vi "Blink Lights.vi"(8 "error in (no error)":errorcluster, 11 "BlinkyLightModel In":refnum<class "BlinkyLightModel.lvclass">) -> (0 "error out":errorcluster, 3 "BlinkyLightModel Out":refnum<class "BlinkyLightModel.lvclass">)   [LabVIEW 2017, in "BlinkyLightModel.lvlib" / "BlinkyLightModel.lvclass"]
uses:
  <vilib>/gpm_packages/@cs/example/Dynamic Viewables/SequenceSteps/BlinkyLightModel/BlinkyLightModel.lvclass
  C:/Program Files/National Instruments/LabVIEW 2017/vi.lib/gpm_packages/@cs/mva-core/Source/IModel/IModel/IModel.lvclass
  C:/Program Files/National Instruments/LabVIEW 2017/vi.lib/ActorFramework/Actor/Actor.lvclass
  <vilib>/gpm_packages/@cs/example/Dynamic Viewables/SequenceSteps/BlinkyLightModel/BlinkyLightModel.lvclass/BlinkyLightModel.ctl
  <vilib>/gpm_packages/@cs/mva-core/Source/IObserver/IObserver/IObserver.lvclass/IObserver.ctl
  <vilib>/gpm_packages/@cs/mva-core/Source/IModel/IModel/IModel.lvclass/IModel.ctl
  <vilib>/gpm_packages/@cs/mva-core/Source/IMediator/PublishRequest/PublishRequest.lvclass/PublishRequest.ctl
  <vilib>/gpm_packages/@cs/mva-core/Source/IMediator/IMediator Messages/Publish Msg/Publish Msg.lvclass/Publish Msg.ctl
  <vilib>/gpm_packages/@cs/actor-framework-messages/Source/RoundTripMessage/RoundTripMessage.lvclass/RoundTripMessage.ctl
  <vilib>/ActorFramework/Message Enqueuer/Message Enqueuer.lvclass/Message Enqueuer.ctl
  <vilib>/ActorFramework/Actor/Actor.lvclass/Actor.ctl
  cb7bf9b9-956b-4f49-b468-f64f0c203643.vi
  <vilib>/gpm_packages/@cs/mva-core/Source/IMediator/IMediator Messages/Publish Msg/Send Pre-Addressed Publish.vi
  <vilib>/gpm_packages/@cs/mva-core/Source/IObserver/IObserver/Read Unique ID.vi
  <vilib>/gpm_packages/@cs/mva-core/Source/IMediator/PublishRequest/Pack Publish Request.vi
  <vilib>/ActorFramework/Message Enqueuer/Init from Existing Queue.vi
  <vilib>/ActorFramework/Message Enqueuer/Enqueue.vi
  <vilib>/gpm_packages/@cs/actor-framework-messages/Source/RoundTripMessage/Return Round-Trip Message.vi
  <vilib>/gpm_packages/@cs/mva-core/Source/IModel/IModel/IModel.lvclass
  C:/Program Files/National Instruments/LabVIEW 2017/vi.lib/gpm_packages/@cs/mva-core/Source/IObserver/IObserver/IObserver.lvclass
  <vilib>/gpm_packages/@cs/mva-core/Source/IMediator/IMediator Messages/Publish Msg/Publish Msg.lvclass
  C:/Program Files/National Instruments/LabVIEW 2017/vi.lib/gpm_packages/@cs/actor-framework-messages/Source/RoundTripMessage/RoundTripMessage.lvclass
  <vilib>/gpm_packages/@cs/actor-framework-messages/Source/RoundTripMessage/RoundTripMessage.lvclass
  C:/Program Files/National Instruments/LabVIEW 2017/vi.lib/ActorFramework/Message/Message.lvclass
  <vilib>/ActorFramework/Stop Msg/Stop Msg.lvclass
  <vilib>/gpm_packages/@cs/example/Dynamic Viewables/SequenceSteps/BlinkyLightModel Messages/Blink Lights Msg/Blink Lights Msg.lvclass
  <vilib>/Utility/error.llb/Error Cluster From Error Code.vi
  <vilib>/ActorFramework/Message Priority Queue/Priority Enqueue.vi
  <vilib>/gpm_packages/@cs/mva-core/Source/IMediator/PublishRequest/PublishRequest.lvclass
  <vilib>/ActorFramework/Message Enqueuer/Message Enqueuer.lvclass
  <vilib>/ActorFramework/Actor/Actor.lvclass
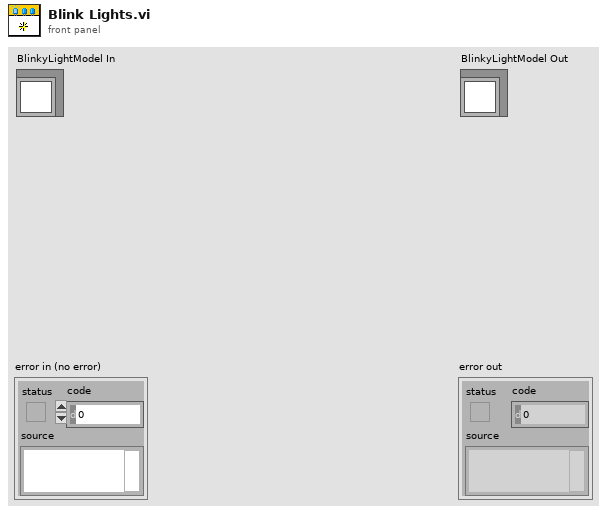
[diagram p1: front panel]
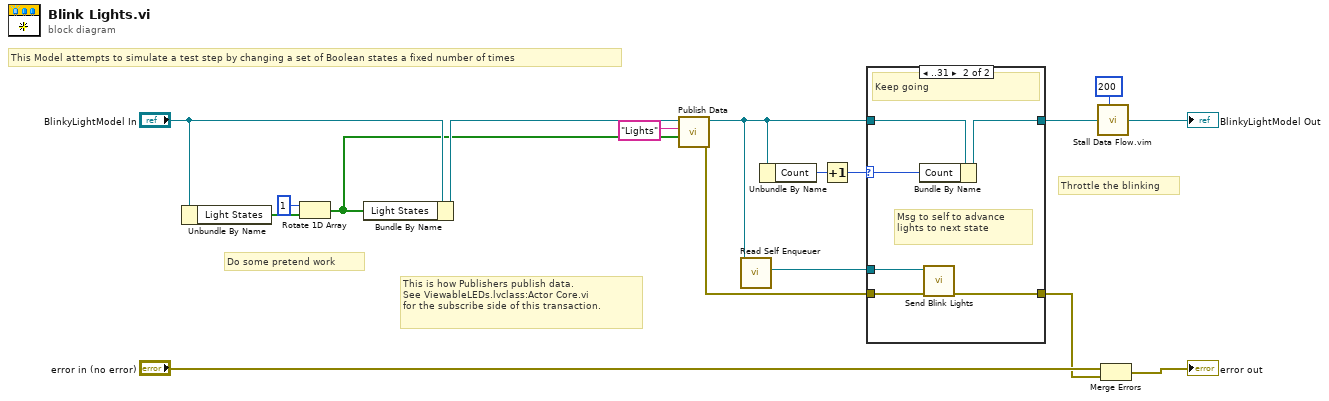
[diagram p0: block diagram]
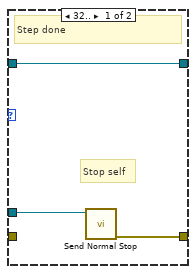
[diagram p2: hidden frame]
diagram:
  # "Do some pretend work"
  # "Throttle the blinking"
  # "This Model attempts to simulate a test step by changing a set of Boolean states a fixed number of times"
  # "This is how Publishers publish data.\nSee ViewableLEDs.lvclass:Actor Core.vi\nfor the subscribe side of this transaction."
  n1 = Unbundle By Name("BlinkyLightModel In") -> ("Light States"=w5:bool[])
  n2 = Rotate 1D Array(1:w5, 2:1 ("n")) -> (0:w2:bool[])
  n3 = Bundle By Name(cluster="BlinkyLightModel In", "Light States"=w2) -> (w4:refnum<class "BlinkyLightModel.lvclass">)
  n4 = call <vilib>:"Publish Data.vi"("Data to Publish"=w2, "Datum Name"="Lights", "IModel in"=w4) -> ("error out"=w15:errorcluster, "IModel out"=w10:refnum<class "BlinkyLightModel.lvclass">)  [unwired: 7 in]
  n5 = call <vilib>:"Read Self Enqueuer.vi"("Actor"=w10) -> ("Self Enqueuer"=w14:refnum<class "Message Enqueuer.lvclass">)  [unwired: 10 in]
  n6 = Unbundle By Name(w10) -> ("Count"=w9:i32)
  n7 = Increment(x=w9) -> (x+1=w8:i32)
  n8 = case shown="..31" w8 {
    selector: w8 -> [_ w21]
    tunnel: w15 -> [_ w26]
    tunnel: w14 -> [w19 w25]
    tunnel: [w18 w24] -> w13
    tunnel: w10 -> [w20 w23]
    tunnel: [w20 w22] -> w7
    frame 32.. {
      # "Stop self"
      # "Step done"
      n9 = call <vilib>:"Send Normal Stop.vi"("Message Enqueuer"=w19) -> ("error out"=w18:errorcluster)  [unwired: 10 in]
    }
    frame ..31 {
      # "Msg to self to advance\nlights to next state"
      # "Keep going"
      n10 = Bundle By Name(cluster=w23, "Count"=w21) -> (w22:refnum<class "BlinkyLightModel.lvclass">)
      n11 = call <vilib>:"Send Blink Lights.vi"("error in (no error)"=w26, "Message Enqueuer"=w25) -> ("error out"=w24:errorcluster)  [unwired: 8 in, 1 out]
    }
  }
  n12 = call "Stall Data Flow.vim"("value in"=w7, "milliseconds to wait"=u32 200) -> ("value out"=→"BlinkyLightModel Out":refnum<class "BlinkyLightModel.lvclass">)  [unwired: 1 out]
  n13 = Merge Errors("error in (no error)", w13) -> (→"error out":errorcluster)
